vi "Z_state.vi"(4 "ZB":bool[](array[boolean])=[FALSE, FALSE], 6 "XB":bool[](array[boolean])=[FALSE, FALSE, FALSE, FALSE, FALSE], 9 "Alarm":bool[](array[boolean])=[FALSE, FALSE], 10 "Z_In":cluster{"Z_Source":T1, "Z_Set_State":T2}={"Z_Source"=enum."hand", "Z_Set_State"=enum."initialization"}, 11 "HE1_Z_state in":refnum<class "HE_Z_state_v2.lvclass">) -> (3 "HE1_Z_state out":refnum<class "HE_Z_state_v2.lvclass">)   [LabVIEW 2019, in "Heating.lvlib" / "HE_Z_state_v2.lvclass"]
uses:
  HE_Z_state_v2.lvclass
  C:/my_projects/projects/Algorithms/Labview/19/Heating/heating1/ZM_state/HE_ZM_state.lvclass
  ctl/Z_source.ctl
  ctl/Z_State.ctl
  ZM_state/HE_ZM_state.lvclass/HE_ZM_state.ctl
  HE_Z_state_v2.lvclass/HE_Z_state_v2.ctl
  ZM_state/HE_ZM_state.lvclass
  C:/my_projects/projects/Algorithms/Labview/19/Sequence/State/State.lvclass
  Sequence/State/State.lvclass
  Heating.lvlib
panel:
  # "XB01 contactor on\nXB02 contactor off\nXB24 local hand on\nheating end\ncooling end"
  # "ZB01 contactor on reg\nZB02 contactor not off reg"
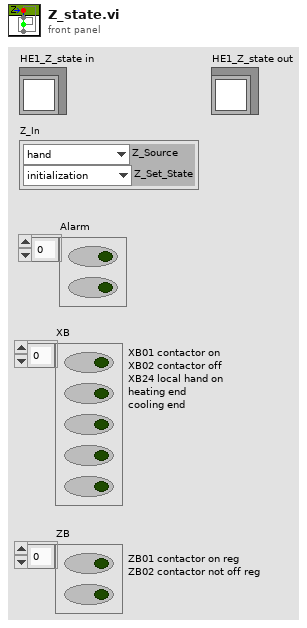
[diagram p1: front panel]
types:
  T1 = typedef "Heating.lvlib/Z_source.ctl" = enum8{"initialize", "local disabled", "local hand", "hand", "auto", "dist"}
  T2 = typedef "Heating.lvlib/Z_State.ctl" = enum8{"initialization", "alarm", "disabled", "not ready", "stop ready", "reserv", "switched off", "reserv2", "switched on", "check", "on min", "decrease out", "on", "increase out", "on max"}
  T3 = typedef "Heating.lvlib/ZM_State.ctl" = enum8{"initialization", "stop", "start_cmd", "contactor_on_cmd", "heating", "on", "stop_cmd", "power_down", "contactor_off_cmd", "cooling", "restart_delay"}
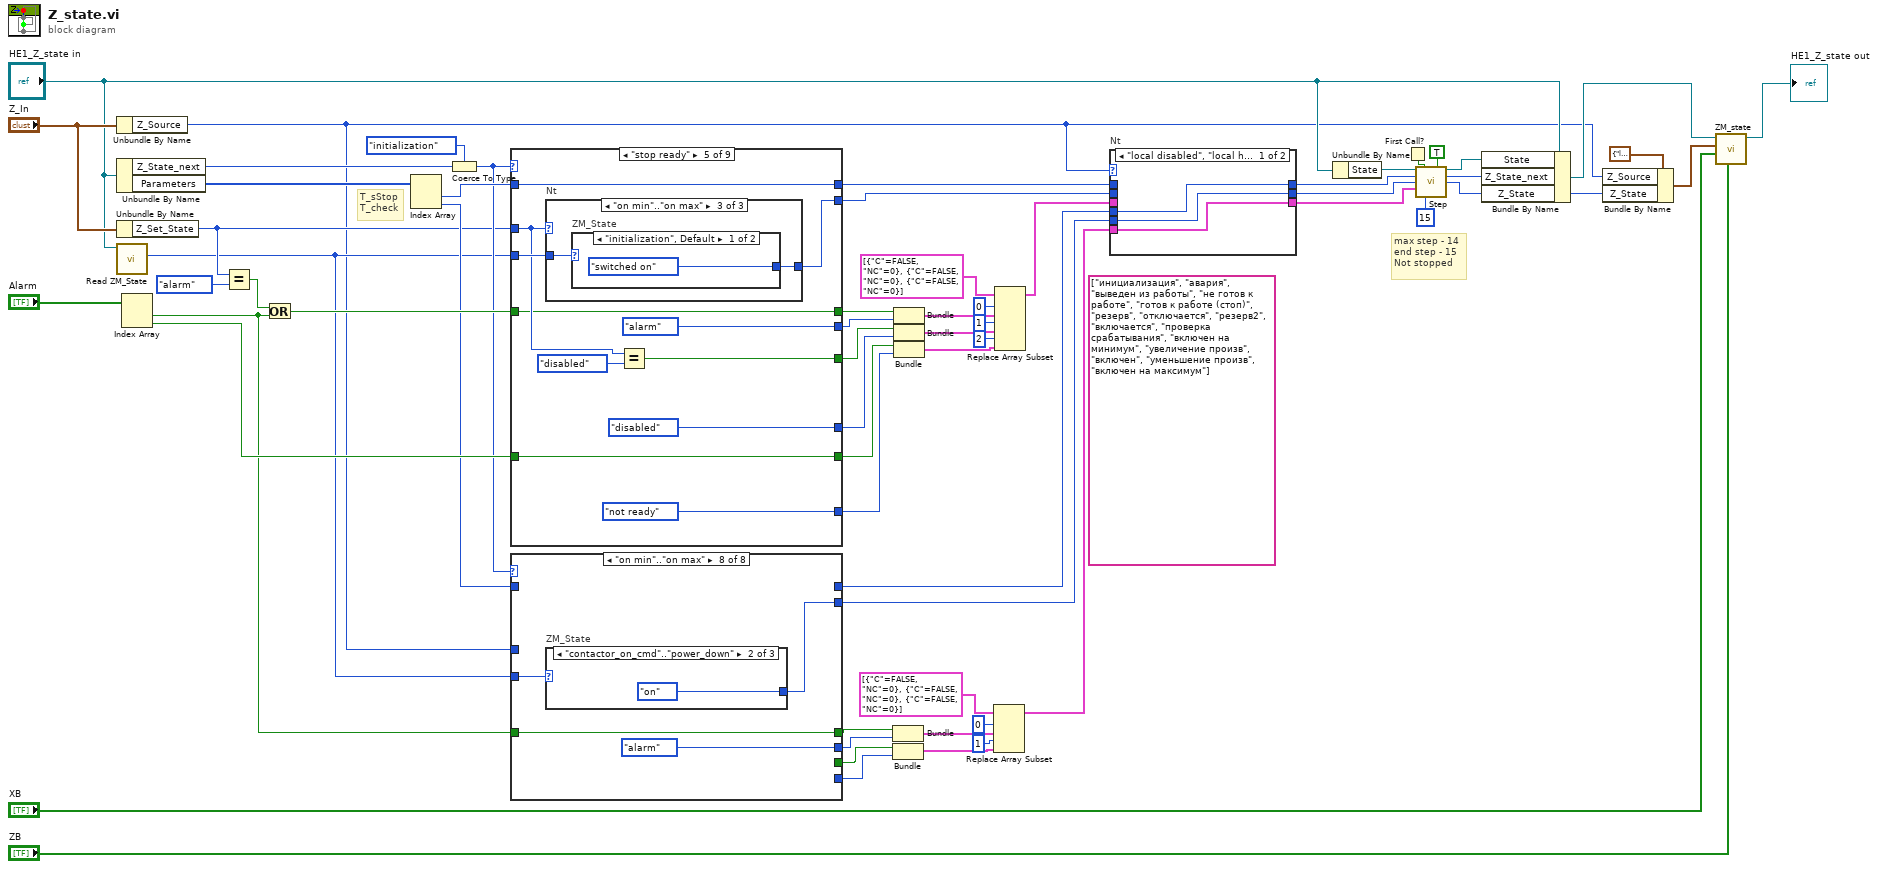
[diagram p0: block diagram]
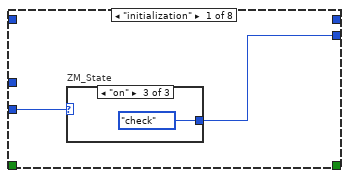
[diagram p2: hidden frame]
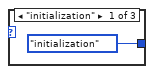
[diagram p3: hidden frame]
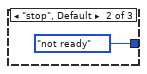
[diagram p4: hidden frame]
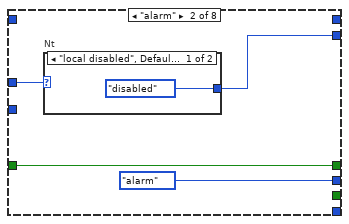
[diagram p5: hidden frame]
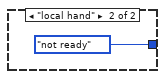
[diagram p6: hidden frame]
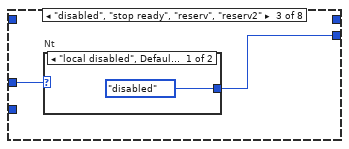
[diagram p7: hidden frame]
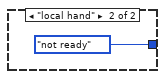
[diagram p8: hidden frame]
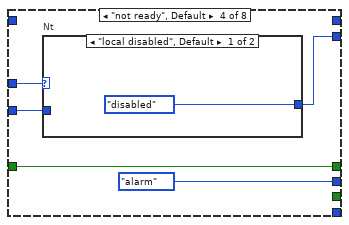
[diagram p9: hidden frame]
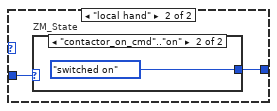
[diagram p10: hidden frame]
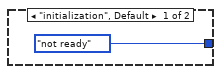
[diagram p11: hidden frame]
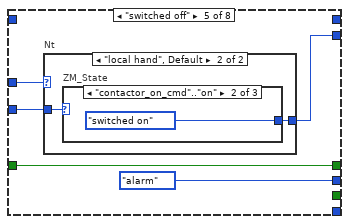
[diagram p12: hidden frame]
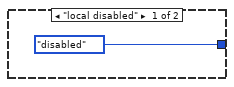
[diagram p13: hidden frame]
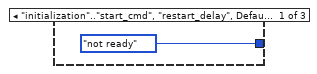
[diagram p14: hidden frame]
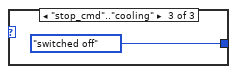
[diagram p15: hidden frame]
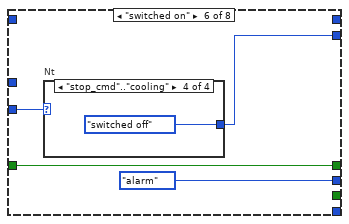
[diagram p16: hidden frame]
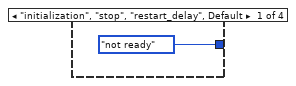
[diagram p17: hidden frame]
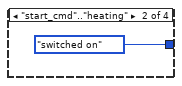
[diagram p18: hidden frame]
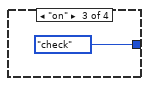
[diagram p19: hidden frame]
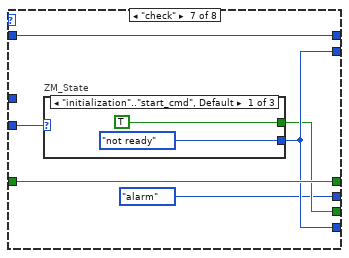
[diagram p20: hidden frame]
diagram:
  (unwired) string[] ["инициализация", "авария", "выведен из работы", "не готов к работе", "готов к работе (стоп)", "резерв", "отключается", "резерв2", "включается", "проверка срабатывания", "включен на минимум", "увеличение произв", "включен", "уменьшение произв", "включен на максимум"]
  # "T_sStop\nT_check"
  # "max step - 14\nend step - 15\nNot stopped"
  n1 = Unbundle By Name("Z_In") -> ("Z_Source"=w1:T1)
  n2 = Unbundle By Name("HE1_Z_state in") -> ("Z_State_next"=w20:T2, "Parameters"=w13:u32[])
  n3 = Unbundle By Name("Z_In") -> ("Z_Set_State"=w21:T2)
  n4 = call "Read ZM_State.vi"("HE_ZM_state in"="HE1_Z_state in") -> ("ZM_State"=w12:T3)  [unwired: 9 in, 1 out]
  n5 = Index Array(array="Alarm") -> (element #1=w27:bool, element #2=w49:bool)  [unwired: 2 in]
  n6 = Equal?(x=w21, y=Z_State."alarm") -> (x = y?=w54:bool)
  n7 = Or(x=w54, y=w27) -> (x .or. y?=w53:bool)
  n8 = Index Array(array=w13) -> (element #1=w50:u32, element #2=w29:u32)  [unwired: 2 in]
  n9 = Coerce To Type(0:w20, 1:Z_State."initialization" ("Z_SetState")) -> (2:w28:T2)
  n10 = case shown="\"stop ready\"" w28 {
    tunnel: w53 -> [_ w70 w77 w85 w95 w115 w127 w143 w158]
    tunnel: w21 -> [w62 w71 w78 w86 w99 w116 w128 w141 w154]
    tunnel: w49 -> [_ _ _ w83 w97 w114 w124 w144 w156]
    tunnel: w50 -> [_ _ _ _ w98 _ _ _ _]
    tunnel: w12 -> [w64 _ _ _ w100 _ w121 w147 _]
    tunnel: [_ _ _ Z_State."not ready" ("Z_SetState") Z_State."not ready" ("Z_SetState") Z_State."not ready" ("Z_SetState") w120 Z_State."switched off" ("Z_SetState") Z_State."switched off" ("Z_SetState")] -> w33
    tunnel: [_ _ _ _ w98 _ _ _ _] -> w14
    tunnel: [_ _ _ w83 w97 w114 w124 w146 w157] -> w32
    tunnel: [_ _ _ _ Z_State."disabled" ("Z_SetState") _ w125 _ _] -> w31
    tunnel: [_ _ _ _ w96 _ w126 _ _] -> w34
    tunnel: [_ Z_State."alarm" ("Z_SetState") Z_State."alarm" ("Z_SetState") Z_State."alarm" ("Z_SetState") Z_State."alarm" ("Z_SetState") Z_State."alarm" ("Z_SetState") Z_State."alarm" ("Z_SetState") Z_State."alarm" ("Z_SetState") Z_State."alarm" ("Z_SetState")] -> w35
    tunnel: [_ w70 w77 w85 w95 w115 w127 w143 w158] -> w36
    tunnel: [w63 w69 w76 w84 w94 w113 w123 w142 w154] -> w15
    frame "initialization" {
      n11 = case "ZM_State" shown="\"on\"" w64 {
        tunnel: [Z_State."initialization" ("Z_SetState") Z_State."not ready" ("Z_SetState") w67] -> w63
        tunnel: w62 -> [_ _ w67]
        frame "initialization" {
        }
        frame "stop", Default {
        }
        frame "on" {
        }
      }
    }
    frame "alarm" {
      n12 = case "Nt" shown="\"disabled\"" w71 {
        tunnel: [Z_State."alarm" ("Z_SetState") Z_State."disabled" ("Z_SetState") Z_State."not ready" ("Z_SetState")] -> w69
        frame "alarm", Default {
        }
        frame "disabled" {
        }
        frame "not ready".."on max" {
        }
      }
    }
    frame "disabled" {
      n13 = case "Nt" shown="\"not ready\"..\"on max\"" w78 {
        tunnel: [Z_State."disabled" ("Z_SetState") Z_State."not ready" ("Z_SetState")] -> w76
        frame "alarm", "disabled", Default {
        }
        frame "not ready".."on max" {
        }
      }
    }
    frame "not ready", Default {
      n14 = case "Nt" shown="\"disabled\"" w86 {
        tunnel: [Z_State."alarm" ("Z_SetState") Z_State."disabled" ("Z_SetState") Z_State."not ready" ("Z_SetState") Z_State."stop ready" ("Z_SetState")] -> w84
        frame "alarm", Default {
        }
        frame "disabled" {
        }
        frame "not ready" {
        }
        frame "stop ready".."on max" {
        }
      }
    }
    frame "stop ready" {
      n15 = case "Nt" shown="\"on min\"..\"on max\"" w99 {
        tunnel: [Z_State."stop ready" ("Z_SetState") w103 w107] -> w94
        tunnel: w100 -> [_ w104 w108]
        frame "stop ready", Default {
        }
        frame "reserv" {
          n16 = case "ZM_State" shown="\"initialization\", Default" w104 {
            tunnel: [Z_State."reserv" ("Z_SetState") Z_State."stop ready" ("Z_SetState")] -> w103
            frame "initialization", Default {
            }
            frame "restart_delay" {
            }
          }
        }
        frame "on min".."on max" {
          n17 = case "ZM_State" shown="\"initialization\", Default" w108 {
            tunnel: [Z_State."switched on" ("Z_SetState") Z_State."stop ready" ("Z_SetState")] -> w107
            frame "initialization", Default {
            }
            frame "restart_delay" {
            }
          }
        }
      }
      n18 = Equal?(x=w99, y=Z_State."disabled") -> (x = y?=w96:bool)
    }
    frame "reserv" {
      n19 = case "Nt" shown="\"check\"..\"on max\"" w116 {
        selector: w116 -> [w117 _ _]
        tunnel: [w117 Z_State."stop ready" ("Z_SetState") Z_State."switched on" ("Z_SetState")] -> w113
        frame "alarm".."not ready", "reserv" {
        }
        frame "stop ready", Default {
        }
        frame "check".."on max" {
        }
      }
    }
    frame "switched off" {
      n20 = case "Nt" shown="\"stop ready\", \"reserv\", \"check\", Default" w128 {
        tunnel: [w134 Z_State."switched on" ("Z_SetState")] -> w123
        tunnel: w121 -> [w135 _]
        frame "stop ready", "reserv", "check", Default {
          n21 = case "ZM_State" shown="\"on\"..\"cooling\"" w135 {
            tunnel: [Z_State."stop ready" ("Z_SetState") Z_State."switched off" ("Z_SetState")] -> w134
            frame "initialization", Default {
            }
            frame "on".."cooling" {
            }
          }
        }
        frame "on min".."on max" {
        }
      }
      n22 = case "ZM_State" shown="\"on\"..\"cooling\"" w121 {
        tunnel: [Z_State."disabled" ("Z_SetState") Z_State."switched off" ("Z_SetState")] -> w125
        frame "initialization", "stop", "restart_delay", Default {
        }
        frame "on".."cooling" {
        }
      }
      n23 = case "ZM_State" shown="\"on\"..\"cooling\"" w121 {
        tunnel: [Z_State."not ready" ("Z_SetState") Z_State."switched off" ("Z_SetState")] -> w120
        frame "initialization", "stop", "restart_delay", Default {
        }
        frame "on".."cooling" {
        }
      }
      n24 = Equal?(x=w128, y=Z_State."disabled") -> (x = y?=w126:bool)
    }
    frame "switched on" {
      n25 = case "ZM_State" shown="\"initialization\", Default" w147 {
        tunnel: [Z_State."switched on" ("Z_SetState") w149] -> w142
        tunnel: w141 -> [_ w149]
        frame "initialization", Default {
        }
        frame "on" {
        }
      }
      n26 = case "Z2" shown="\"disabled\"..\"reserv\", Default" w141 {
        tunnel: [FALSE TRUE] -> w145
        frame "check".."on max" {
        }
        frame "disabled".."reserv", Default {
        }
      }
      n27 = Or(x=w145, y=w144) -> (x .or. y?=w146:bool)
    }
    frame "check".."on max" {
      n28 = case "Z2" shown="\"disabled\"..\"reserv\", Default" w154 {
        tunnel: [FALSE TRUE] -> w155
        frame "check".."on max" {
        }
        frame "disabled".."reserv", Default {
        }
      }
      n29 = Or(x=w155, y=w156) -> (x .or. y?=w157:bool)
    }
  }
  n30 = case shown="\"on min\"..\"on max\"" w28 {
    tunnel: w27 -> [_ w169 _ w180 w190 w200 w210 w220]
    tunnel: w1 -> [_ w168 w173 w179 w189 _ _ _]
    tunnel: w12 -> [w162 _ _ w177 w188 w199 w209 w218]
    tunnel: [_ _ _ _ _ _ w208 _] -> w23
    tunnel: [_ _ _ _ _ _ w207 _] -> w24
    tunnel: [_ Z_State."alarm" ("Z_SetState") _ Z_State."alarm" ("Z_SetState") Z_State."alarm" ("Z_SetState") Z_State."alarm" ("Z_SetState") Z_State."alarm" ("Z_SetState") Z_State."alarm" ("Z_SetState")] -> w25
    tunnel: [_ w169 _ w180 w190 w200 w210 w220] -> w26
    tunnel: [w161 w167 w172 w178 w187 w198 w208 w217] -> w16
    tunnel: w29 -> [_ _ _ _ _ _ w206 _]
    tunnel: [_ _ _ _ _ _ w206 _] -> w17
    frame "initialization" {
      n31 = case "ZM_State" shown="\"on\"" w162 {
        tunnel: [Z_State."initialization" ("Z_SetState") Z_State."not ready" ("Z_SetState") Z_State."check" ("Z_SetState")] -> w161
        frame "initialization" {
        }
        frame "stop", Default {
        }
        frame "on" {
        }
      }
    }
    frame "alarm" {
      n32 = case "Nt" shown="\"local disabled\", Default" w168 {
        tunnel: [Z_State."disabled" ("Z_SetState") Z_State."not ready" ("Z_SetState")] -> w167
        frame "local disabled", Default {
        }
        frame "local hand" {
        }
      }
    }
    frame "disabled", "stop ready", "reserv", "reserv2" {
      n33 = case "Nt" shown="\"local disabled\", Default" w173 {
        tunnel: [Z_State."disabled" ("Z_SetState") Z_State."not ready" ("Z_SetState")] -> w172
        frame "local disabled", Default {
        }
        frame "local hand" {
        }
      }
    }
    frame "not ready", Default {
      n34 = case "Nt" shown="\"local disabled\", Default" w179 {
        tunnel: [Z_State."disabled" ("Z_SetState") w183] -> w178
        tunnel: w177 -> [_ w182]
        frame "local disabled", Default {
        }
        frame "local hand" {
          n35 = case "ZM_State" shown="\"contactor_on_cmd\"..\"on\"" w182 {
            tunnel: [Z_State."not ready" ("Z_SetState") Z_State."switched on" ("Z_SetState")] -> w183
            frame "initialization", Default {
            }
            frame "contactor_on_cmd".."on" {
            }
          }
        }
      }
    }
    frame "switched off" {
      n36 = case "Nt" shown="\"local hand\", Default" w189 {
        tunnel: [Z_State."disabled" ("Z_SetState") w192] -> w187
        tunnel: w188 -> [_ w193]
        frame "local disabled" {
        }
        frame "local hand", Default {
          n37 = case "ZM_State" shown="\"contactor_on_cmd\"..\"on\"" w193 {
            tunnel: [Z_State."not ready" ("Z_SetState") Z_State."switched on" ("Z_SetState") Z_State."switched off" ("Z_SetState")] -> w192
            frame "initialization".."start_cmd", "restart_delay", Default {
            }
            frame "contactor_on_cmd".."on" {
            }
            frame "stop_cmd".."cooling" {
            }
          }
        }
      }
    }
    frame "switched on" {
      n38 = case "Nt" shown="\"stop_cmd\"..\"cooling\"" w199 {
        tunnel: [Z_State."not ready" ("Z_SetState") Z_State."switched on" ("Z_SetState") Z_State."check" ("Z_SetState") Z_State."switched off" ("Z_SetState")] -> w198
        frame "initialization", "stop", "restart_delay", Default {
        }
        frame "start_cmd".."heating" {
        }
        frame "on" {
        }
        frame "stop_cmd".."cooling" {
        }
      }
    }
    frame "check" {
      n39 = case "ZM_State" shown="\"initialization\"..\"start_cmd\", Default" w209 {
        tunnel: [Z_State."not ready" ("Z_SetState") Z_State."on" ("Z_SetState") Z_State."switched off" ("Z_SetState")] -> w208
        tunnel: [TRUE FALSE TRUE] -> w207
        frame "initialization".."start_cmd", Default {
        }
        frame "contactor_on_cmd".."power_down" {
        }
        frame "contactor_off_cmd".."restart_delay" {
        }
      }
    }
    frame "on min".."on max" {
      n40 = case "ZM_State" shown="\"contactor_on_cmd\"..\"power_down\"" w218 {
        tunnel: [Z_State."not ready" ("Z_SetState") Z_State."on" ("Z_SetState") Z_State."switched off" ("Z_SetState")] -> w217
        frame "initialization".."start_cmd", Default {
        }
        frame "contactor_on_cmd".."power_down" {
        }
        frame "contactor_off_cmd".."restart_delay" {
        }
      }
    }
  }
  n41 = Bundle("Alarm"=w26, "Z_SetState"=w25) -> (w39:cluster{"Alarm":bool, "Z_SetState":T2})  [unwired: 1 in]
  n42 = Bundle(w24, "Z_SetState"=w23) -> (w41:cluster{bool, "Z_SetState":T2})  [unwired: 1 in]
  n43 = Bundle(w36, "Z_SetState"=w35) -> (w46:cluster{bool, "Z_SetState":T2})  [unwired: 1 in]
  n44 = Bundle(w34, "Z_SetState"=w31) -> (w43:cluster{bool, "Z_SetState":T2})  [unwired: 1 in]
  n45 = Bundle("Alarm"=w32, "Z_SetState"=w33) -> (w42:cluster{"Alarm":bool, "Z_SetState":T2})  [unwired: 1 in]
  n46 = Replace Array Subset(array=cluster{"C":bool, "NC":u32}[] [{"C"=FALSE, "NC"=0}, {"C"=FALSE, "NC"=0}, {"C"=FALSE, "NC"=0}] ("appended array"), new element #1=w39, index #1=0 ("index"), new element #2=w41, index #2=1 ("index")) -> (w19:cluster{"C":bool, "NC":u32}[])
  n47 = Replace Array Subset(array=cluster{"C":bool, "NC":u32}[] [{"C"=FALSE, "NC"=0}, {"C"=FALSE, "NC"=0}, {"C"=FALSE, "NC"=0}] ("appended array"), new element #1=w46, index #1=0 ("index"), new element #2=w43, index #2=1 ("index"), new element #3=w42, index #3=2 ("index")) -> (w18:cluster{"C":bool, "NC":u32}[])
  n48 = case "Nt" shown="\"local disabled\", \"local hand\"" w1 {
    tunnel: w15 -> [_ w229]
    tunnel: w18 -> [_ w228]
    tunnel: [w225 w229] -> w58
    tunnel: [w226 w228] -> w59
    tunnel: w16 -> [w225 _]
    tunnel: w19 -> [w226 _]
    tunnel: w14 -> [_ w227]
    tunnel: [w224 w227] -> w57
    tunnel: w17 -> [w224 _]
    frame "local disabled", "local hand" {
    }
    frame "hand".."dist", Default {
    }
  }
  n49 = Unbundle By Name("HE1_Z_state in") -> ("State"=w9:refnum<class "State.lvclass">)
  n50 = First Call?() -> (First Call?: T/F=w61:bool)
  n51 = call "Step.vi"("State in"=w9, "Reset"=w61, "Start in"=TRUE ("Start"), "t"=w57, "Nt"=w58, "C_table"=w59, "N end step"=u32 15) -> ("State out"=w7:refnum<class "State.lvclass">, "N next"=w60:u32, "N curr"=w6:u32)  [unwired: 5 in, 1 out]
  n52 = Bundle By Name(cluster="HE1_Z_state in", "State"=w7, "Z_State_next"=w60, "Z_State"=w6) -> (w5:refnum<class "HE_Z_state_v2.lvclass">)
  n53 = Bundle By Name(cluster=cluster{"Z_Source":T1, "Z_State":T2} {"Z_Source"=enum."local disabled", "Z_State"=enum."alarm"} ("Z_In"), "Z_Source"=w1, "Z_State"=w6) -> (w10:cluster{"Z_Source":T1, "Z_State":T2})
  n54 = call "ZM_state.vi"("ZB"="ZB", "XB"="XB", "Z_In"=w10, "ZM_state in"=w5) -> ("ZM_state out"=→"HE1_Z_state out":refnum<class "HE_Z_state_v2.lvclass">)  [unwired: 7 in]
